vi "Serialize - JSON.vi"(8 "error in":errorcluster, 11 "TECData in":refnum<class "TECData.lvclass">) -> (0 "error out":errorcluster, 2 "Serialized JSON":string, 3 "TECData out":refnum<class "TECData.lvclass">)   [LabVIEW 2014, in "TE Cooler.lvlib" / "TECData.lvclass"]
uses:
  TECData.lvclass
  reusable/Data/Data.lvclass/Data.ctl
  TECData.lvclass/TECData.ctl
  reusable/Data/Read Data ID.vi
  Data Access/Read Input 1.vi
  Data Access/Read Input 2.vi
  Data Access/Read Power.vi
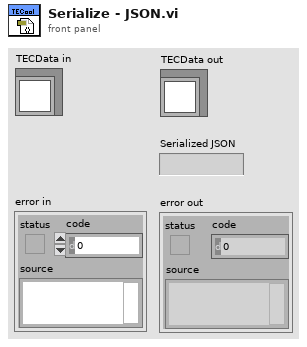
[diagram p1: front panel]
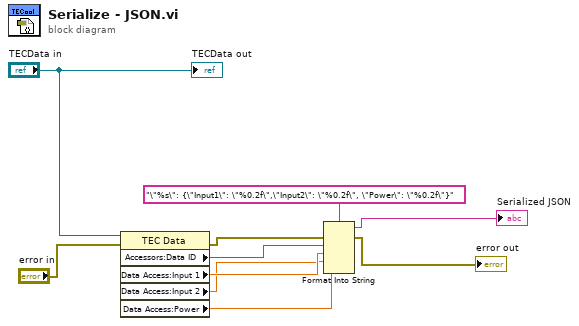
[diagram p0: block diagram]
diagram:
  n1 = property class="TEC Data"(reference="TECData in", error in="error in") -> (error out=w7:errorcluster, "Accessors:Data ID"=w6:string, "Data Access:Input 1"=w5:sgl, "Data Access:Input 2"=w4:sgl, "Data Access:Power"=w3:sgl)  [unwired: 1 out]
  n2 = Format Into String(format string="\"%s\": {\"Input1\": \"%0.2f\",\"Input2\": \"%0.2f\", \"Power\": \"%0.2f\"}", error in=w7, w6, w5, w4, w3) -> (resulting string=→"Serialized JSON":string, error out=→"error out":errorcluster)  [unwired: 1 in]
  "TECData out" <- "TECData in"
